vi "oa_SCL Calc Text Rect.vi"(5 "[user-specified font]":T3, 7 "desired font(Application)":T2(ring)=enum."Application Font", 11 "xy axis":T4={"x minimum"=0.0, "x maximum"=0.0, "x log?"=FALSE, "x precision"=1, "x format"=enum."Decimal", "y minimum"=0.0, "y maximum"=0.0, "y log?"=FALSE, "y precision"=1, "y format"=enum."Decimal"} {"x minimum" format="%.2f"; "x maximum" format="%.2f"; "y minimum" format="%.2f"; "y maximum" format="%.2f"}) -> (2 "y rect":T1, 3 "x rect":T1)   [LabVIEW 2017]
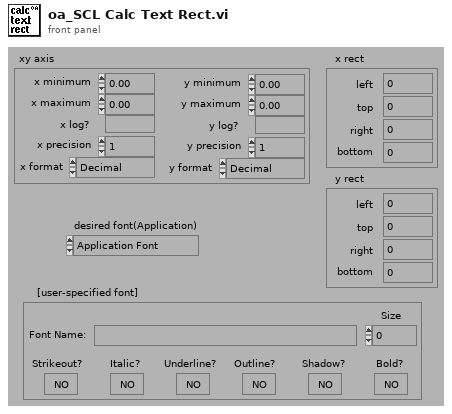
[diagram p1: front panel]
types:
  T1 = cluster{"left":i16, "top":i16, "right":i16, "bottom":i16}
  T2 = enum16{"User-specified Font", "Application Font", "System Font", "Dialog Font"}
  T3 = cluster{"Font Name:":string, "Size":i16, "Strikeout?":bool, "Italic?":bool, "Underline?":bool, "Outline?":bool, "Shadow?":bool, "Bold?":bool}
  T4 = cluster{"x minimum":dbl, "x maximum":dbl, "x log?":bool, "x precision":u8, "x format":enum8{"Decimal", "Scientific", "Engineering", "Binary", "Octal", "Hex"}, "y minimum":dbl, "y maximum":dbl, "y log?":bool, "y precision":u8, "y format":enum8{"Decimal", "Scientific", "Engineering", "Binary", "Octal", "Hex"}}
  T5 = enum8{"Decimal", "Scientific", "Engineering", "Binary", "Octal", "Hex"}
  T6 = cluster{"y format":enum8{"Decimal", "Scientific", "Engineering", "Binary", "Octal", "Hex"}, "y precision":u8}
  T7 = cluster{"x format":enum8{"Decimal", "Scientific", "Engineering", "Binary", "Octal", "Hex"}, "x precision":u8}
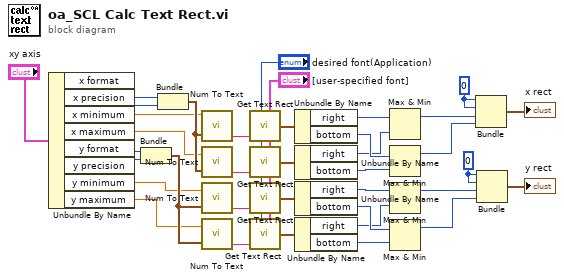
[diagram p0: block diagram]
diagram:
  w12 = i16 0
  w15 = i16 0
  n1 = Unbundle By Name("xy axis") -> ("x format"=w3:T5, "x precision"=w4:u8, "x minimum"=w35:dbl, "x maximum"=w34:dbl, "y format"=w2:T5, "y precision"=w1:u8, "y minimum"=w33:dbl, "y maximum"=w32:dbl)
  n2 = Bundle("y format"=w2, "y precision"=w1) -> (w37:T6)  [unwired: 1 in]
  n3 = Bundle("x format"=w3, "x precision"=w4) -> (w36:T7)  [unwired: 1 in]
  n4 = call <vilib>:"Num To Text.vi"("fmt and prec"=w36, "number"=w35) -> ("numeric string"=w31:string)
  n5 = call <vilib>:"Num To Text.vi"("fmt and prec"=w36, "number"=w34) -> ("numeric string"=w30:string)
  n6 = call <vilib>:"Num To Text.vi"("fmt and prec"=w37, "number"=w33) -> ("numeric string"=w29:string)
  n7 = call <vilib>:"Num To Text.vi"("fmt and prec"=w37, "number"=w32) -> ("numeric string"=w28:string)
  n8 = call <vilib>:"Get Text Rect.vi"("desired font(Application)"="desired font(Application)", "text"=w31, "[user-specified font]"="[user-specified font]") -> ("rect"=w27:T1)  [unwired: 6 in]
  n9 = call <vilib>:"Get Text Rect.vi"("desired font(Application)"="desired font(Application)", "text"=w30, "[user-specified font]"="[user-specified font]") -> ("rect"=w26:T1)  [unwired: 6 in]
  n10 = call <vilib>:"Get Text Rect.vi"("desired font(Application)"="desired font(Application)", "text"=w29, "[user-specified font]"="[user-specified font]") -> ("rect"=w25:T1)  [unwired: 6 in]
  n11 = call <vilib>:"Get Text Rect.vi"("desired font(Application)"="desired font(Application)", "text"=w28, "[user-specified font]"="[user-specified font]") -> ("rect"=w24:T1)  [unwired: 6 in]
  n12 = Unbundle By Name(w27) -> ("right"=w23:i16, "bottom"=w21:i16)
  n13 = Unbundle By Name(w26) -> ("right"=w20:i16, "bottom"=w19:i16)
  n14 = Unbundle By Name(w25) -> ("right"=w22:i16, "bottom"=w17:i16)
  n15 = Unbundle By Name(w24) -> ("right"=w16:i16, "bottom"=w18:i16)
  n16 = Max & Min(x=w23, y=w20) -> (max(x,y)=w14:i16)  [unwired: 1 out]
  n17 = Max & Min(x=w21, y=w19) -> (max(x,y)=w13:i16)  [unwired: 1 out]
  n18 = Max & Min(x=w22, y=w16) -> (max(x,y)=w11:i16)  [unwired: 1 out]
  n19 = Max & Min(x=w17, y=w18) -> (max(x,y)=w10:i16)  [unwired: 1 out]
  n20 = Bundle(w15, w15, "right"=w14, "bottom"=w13) -> (→"x rect":cluster{i16, i16, "right":i16, "bottom":i16})  [unwired: 1 in]
  n21 = Bundle(w12, w12, "right"=w11, "bottom"=w10) -> (→"y rect":cluster{i16, i16, "right":i16, "bottom":i16})  [unwired: 1 in]
